vi "Periodic Tasks.vi"(8 "error in":errorcluster) -> ()   [LabVIEW 2020]
doc: "This VI runs in parallel to other tasks. It can contain as many user-defined periodic loops as you need. These can carry out PID or other sorts of timed response."
uses:
  <vilib>/Rock Robotics/WPI/Compressor/WPI_CompressorFeedbackMode.ctl
  <vilib>/Rock Robotics/WPI/Utilities/WPI_GetSetVariantRefNum.vi
panel:
  out "Feedback Configuration":T2={"Feedback Sensor"=enum."Digital Only", "Max Pressure (PSI)"=0.0, "Min Pressure (PSI)"=0.0}
  out "Compressor Running":bool
  out "Enabled":bool
  out "Pressure Sensors":T3
  out "Analog  Sensors":cluster{"Analog 0 (V)":dbl, "Analog 1 (V)":dbl}
  # "e"
  # "e"
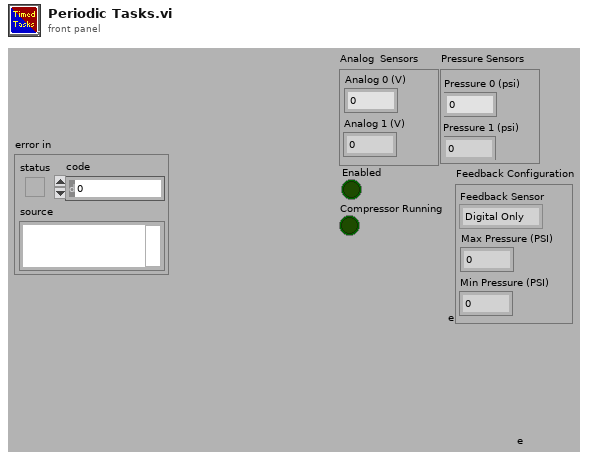
[diagram p1: front panel]
types:
  T1 = typedef "WPI_CompressorFeedbackMode.ctl" = enum16{"Analog Only", "Digital Only", "Hybrid"}
  T2 = cluster{"Feedback Sensor":T1, "Max Pressure (PSI)":dbl, "Min Pressure (PSI)":dbl}
  T3 = cluster{"Pressure 0 (psi)":dbl, "Pressure 1 (psi)":dbl}
  T4 = typedef "WPI_CompressorDevRef.ctl" = cluster{"DevStatus":errorcluster, "Pneumatics Control Module":u8}
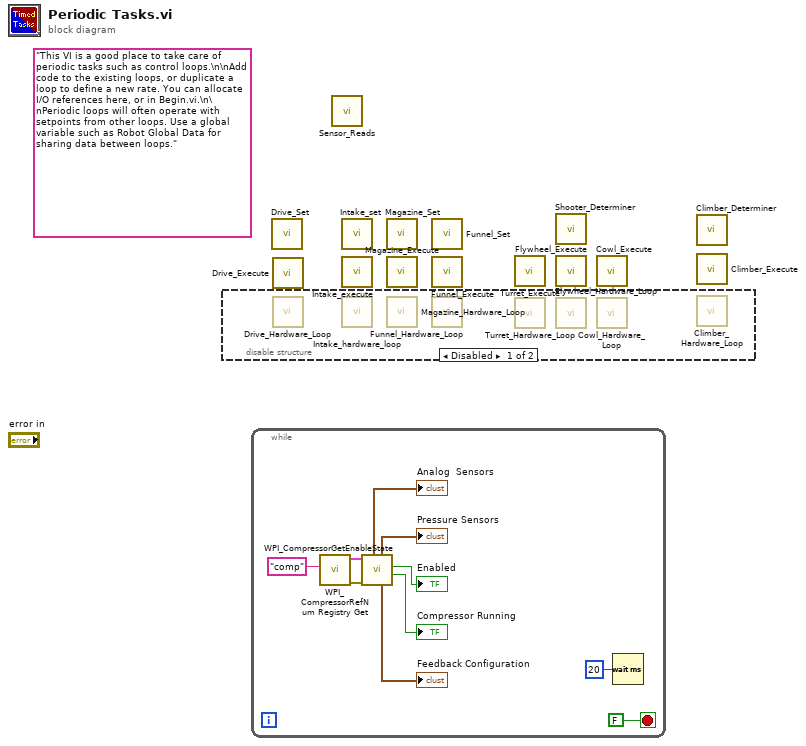
[diagram p0: block diagram]
diagram:
  (unwired) "This VI is a good place to take care of periodic tasks such as control loops.\n\nAdd code to the existing loops, or duplicate a loop to define a new rate. You can allocate I/O references here, or in Begin.vi.\n\nPeriodic loops will often operate with setpoints from other loops. Use a global variable such as Robot Global Data for sharing data between loops."
  n1 = disable-structure shown="Disabled" {
    frame Disabled {
      n2 = call "Drive_Hardware_Loop.vi"() -> ()  [unwired: 12 in]
      n3 = call "Intake_hardware_loop.vi"() -> ()  [unwired: 12 in]
      n4 = call "Magazine_Hardware_Loop.vi"() -> ()  [unwired: 12 in]
      n5 = call "Funnel_Hardware_Loop.vi"() -> ()  [unwired: 12 in]
      n6 = call "Turret_Hardware_Loop.vi"() -> ()  [unwired: 12 in]
      n7 = call "Flywheel_Hardware_Loop.vi"() -> ()  [unwired: 12 in]
      n8 = call "Cowl_Hardware_Loop.vi"() -> ()  [unwired: 12 in]
      n9 = call "Climber_Hardware_Loop.vi"() -> ()  [unwired: 12 in]
    }
    frame Enabled {
    }
  }
  n10 = while {
    stop <- FALSE stop-if-true
    n11 = call <vilib>:"WPI_CompressorRefNum Registry Get.vi"("refnum name"="comp") -> ("error out"=w8:errorcluster, "CompressorDevRef"=w9:T4)  [unwired: 9 in]
    n12 = call <vilib>:"WPI_CompressorGetEnableState.vi"("error in (no error)"=w8, "CompressorDevRef"=w9) -> ("Compressor Running"=→"Compressor Running":bool, "Enabled"=→"Enabled":bool, "Feedback Configuration"=→"Feedback Configuration":T2, "Pressure Sensors"=→"Pressure Sensors":T3, "Analog  Sensors"=→"Analog  Sensors":cluster{"Analog 0 (V)":dbl, "Analog 1 (V)":dbl})  [unwired: 3 in, 2 out]
    n13 = Wait (ms)(milliseconds to wait=u32 20) -> ()  [unwired: 1 out]
  }
  n14 = call "Drive_Set.vi"() -> ()  [unwired: 12 in]
  n15 = call "Drive_Execute.vi"() -> ()  [unwired: 12 in]
  n16 = call "Sensor_Reads.vi"() -> ()  [unwired: 12 in]
  n17 = call "Intake_set.vi"() -> ()  [unwired: 12 in]
  n18 = call "Intake_execute.vi"() -> ()  [unwired: 12 in]
  n19 = call "Magazine_Set.vi"() -> ()  [unwired: 12 in]
  n20 = call "Magazine_Execute.vi"() -> ()  [unwired: 12 in]
  n21 = call "Funnel_Set.vi"() -> ()  [unwired: 12 in]
  n22 = call "Funnel_Execute.vi"() -> ()  [unwired: 12 in]
  n23 = call "Turret_Execute.vi"() -> ()  [unwired: 12 in]
  n24 = call "Shooter_Determiner.vi"() -> ()  [unwired: 12 in]
  n25 = call "Flywheel_Execute.vi"() -> ()  [unwired: 12 in]
  n26 = call "Cowl_Execute.vi"() -> ()  [unwired: 12 in]
  n27 = call "Climber_Determiner.vi"() -> ()  [unwired: 12 in]
  n28 = call "Climber_Execute.vi"() -> ()  [unwired: 12 in]
